vi "SV Signal Property Node.vi"   [LabVIEW 2017]
doc: "Use this property node to configure properties of the signal. Select the property to configure from a list that appears when you click on the property name.\n\nYou can use multple property nodes to set multiple properties or drag-extend the property node to expose multiple property terminals."
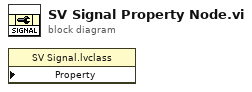
[diagram p0: block diagram]
diagram:
  n1 = property class="SV Signal.lvclass" props=[]() -> ()  [unwired: 3 in, 2 out]
